vi "Device Identity.vi"(8 "error in (no error)":errorcluster, 11 "VisaComms in":refnum<class "VisaComms.lvclass">) -> (0 "error out":errorcluster, 2 "Identity":T1, 3 "VisaComms out":refnum<class "VisaComms.lvclass">)   [LabVIEW 2024, in "CTI.lvlib" / "VisaComms.lvclass"]
uses:
  VisaComms.lvclass
  Identity.ctl
  VisaComms.lvclass/VisaComms.ctl
  Clean Visa Errors.vi
  CTI.lvlib
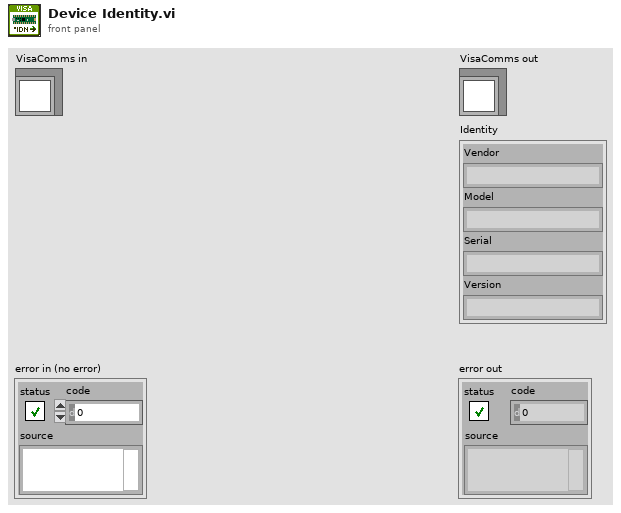
[diagram p1: front panel]
types:
  T1 = typedef "CTI.lvlib/Identity.ctl" = cluster{"Vendor":string, "Model":string, "Serial":string, "Version":string}
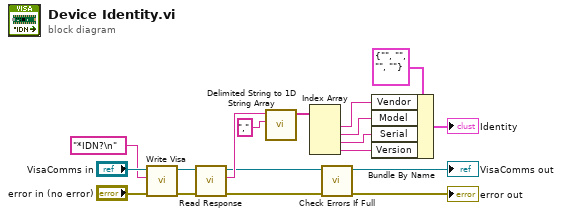
[diagram p0: block diagram]
diagram:
  n1 = call "Write Visa.vi"("error in (no error)"="error in (no error)", "write buffer"="*IDN?\n", "VisaComms in"="VisaComms in") -> ("error out"=w15:errorcluster, "VisaComms out"=w14:refnum<class "VisaComms.lvclass">)  [unwired: 6 in, 1 out]
  n2 = call "Read Response.vi"("error in (no error)"=w15, "VisaComms in"=w14) -> ("error out"=w13:errorcluster, "Response"=w10:string, "VisaComms out"=w2:refnum<class "VisaComms.lvclass">)  [unwired: 6 in, 1 out]
  n3 = call <vilib>:"Delimited String to 1D String Array.vi"("delimiter"=",", "delimited string"=w10) -> ("string array"=w8:string[])  [unwired: 9 in]
  n4 = Index Array(array=w8) -> (element #1=w7:string, element #2=w6:string, element #3=w5:string, element #4=w4:string)  [unwired: 4 in]
  n5 = call "Check Errors If Full.vi"("error in (no error)"=w13, "VisaComms in"=w2) -> ("error out"=→"error out":errorcluster, "VisaComms out"=→"VisaComms out":refnum<class "VisaComms.lvclass">)  [unwired: 8 in]
  n6 = Bundle By Name(cluster=T1 {"Vendor"="", "Model"="", "Serial"="", "Version"=""} ("Identity"), "Vendor"=w7, "Model"=w6, "Serial"=w5, "Version"=w4) -> (→"Identity":T1)
